vi "Is Pending Operation.vi"(8 "error in":errorcluster, 11 "Remote Operation Abstract":refnum<class "Remote Operation Abstract.lvclass">) -> (0 "error out":errorcluster, 2 "Pending?":bool, 3 "dup Remote Operation Abstract":refnum<class "Remote Operation Abstract.lvclass">)   [LabVIEW 2018, in "Remote Operation Abstract.lvlib" / "Remote Operation Abstract.lvclass"]
uses:
  Remote Operation Abstract.lvclass
  Remote Operation Abstract.lvclass/Remote Operation Abstract.ctl
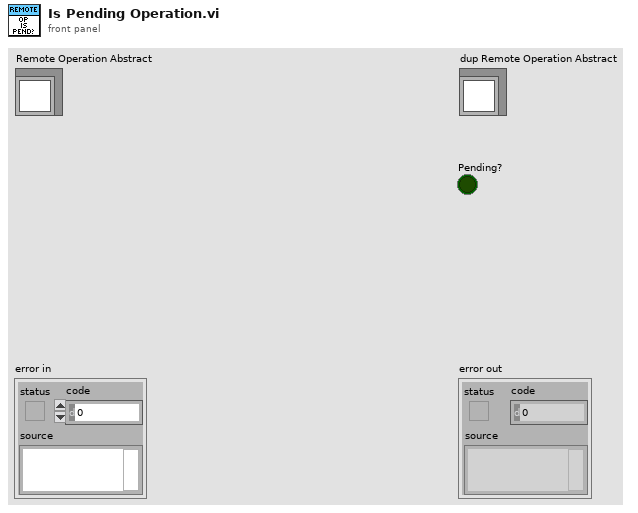
[diagram p1: front panel]
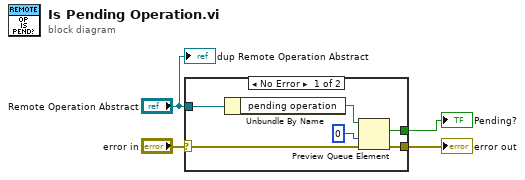
[diagram p0: block diagram]
diagram:
  n1 = case shown="No Error" "error in" {
    selector: "error in" -> [w9 w11]
    tunnel: [w8 w11] -> w3
    tunnel: "Remote Operation Abstract" -> [w10 _]
    tunnel: [w6 _] -> w1
    frame No Error {
      n2 = Unbundle By Name(w10) -> ("pending operation"=w7:refnum<queue>)
      n3 = Preview Queue Element(queue=w7, timeout in ms (-1)=0, error in (no error)=w9) -> (element=w6:bool, error out=w8:errorcluster)  [unwired: 2 out]
    }
    frame Error {
    }
  }
  "error out" <- w3
  "Pending?" <- w1
  "dup Remote Operation Abstract" <- "Remote Operation Abstract"
